vi "cam-draw-target-cross-hair.vi"(11 "Refnum in":T1) -> (3 "Refnum out":T1)   [LabVIEW 2020]
uses:
  <vilib>/vision/Image Controls.llb/IMAQ Image.ctl
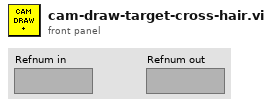
[diagram p1: front panel]
types:
  T1 = typedef "IMAQ Image.ctl" = refnum<image>
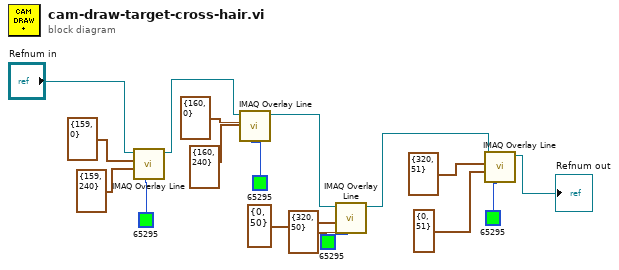
[diagram p0: block diagram]
diagram:
  n1 = call "IMAQ Overlay Line"("Color"=u32 65295, "End Point"=cluster{"X":i32, "Y":i32} {"X"=159, "Y"=240}, "Start Point"=cluster{"X":i32, "Y":i32} {"X"=159, "Y"=0}, "Image"="Refnum in") -> ("Image Out"=w5:T1)  [unwired: 6 in, 1 out]
  n2 = call "IMAQ Overlay Line"("Color"=u32 65295, "End Point"=cluster{"X":i32, "Y":i32} {"X"=160, "Y"=240}, "Start Point"=cluster{"X":i32, "Y":i32} {"X"=160, "Y"=0}, "Image"=w5) -> ("Image Out"=w10:T1)  [unwired: 6 in, 1 out]
  n3 = call "IMAQ Overlay Line"("Color"=u32 65295, "End Point"=cluster{"X":i32, "Y":i32} {"X"=0, "Y"=50}, "Start Point"=cluster{"X":i32, "Y":i32} {"X"=320, "Y"=50}, "Image"=w10) -> ("Image Out"=w9:T1)  [unwired: 6 in, 1 out]
  n4 = call "IMAQ Overlay Line"("Color"=u32 65295, "End Point"=cluster{"X":i32, "Y":i32} {"X"=0, "Y"=51}, "Start Point"=cluster{"X":i32, "Y":i32} {"X"=320, "Y"=51}, "Image"=w9) -> ("Image Out"=→"Refnum out":T1)  [unwired: 6 in, 1 out]
